vi "SSB.vi"() -> ()   [LabVIEW 2018]
uses:
  <vilib>/express/express analysis/Spectral/Block/exnSpectralBlock spectral measurements RMS poly.vi
  <vilib>/express/express analysis/Spectral/Block/exnSpectralBlock spectral measurements RMS DDT.vi
  <vilib>/express/express analysis/Spectral/XNode/ExpressSpectralMeasurementsBlockNode.xnode
panel:
  out "USB 2":dynamicdata(graph)
  out "Waveform Graph":dynamicdata(graph)
  out "LSB 2":dynamicdata(graph)
  out "USB":dynamicdata(graph)
  out "LSB":dynamicdata(graph)
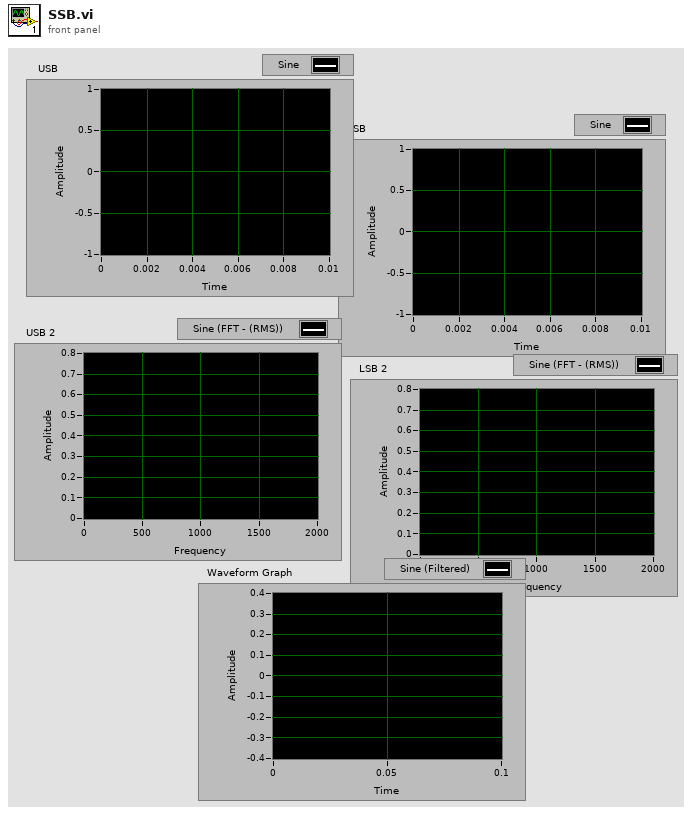
[diagram p1: front panel]
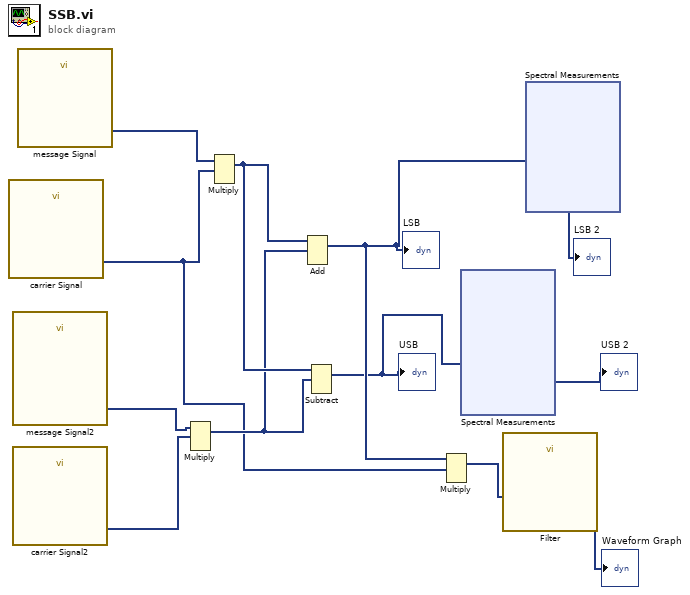
[diagram p0: block diagram]
diagram:
  n1 = call "carrier Signal"() -> ("Sine"=w7:dynamicdata)  [unwired: 14 in, 1 out]
  n2 = call "message Signal2"() -> ("Sine"=w11:dynamicdata)  [unwired: 14 in, 1 out]
  n3 = call "carrier Signal2"() -> ("Sine"=w10:dynamicdata)  [unwired: 14 in, 1 out]
  n4 = call "message Signal"() -> ("Sine"=w12:dynamicdata)  [unwired: 14 in, 1 out]
  n5 = Multiply(1:w10, 2:w11) -> (0:w8:dynamicdata)  [unwired: 1 in, 1 out]
  n6 = Multiply(1:w7, 2:w12) -> (0:w9:dynamicdata)  [unwired: 1 in, 1 out]
  n7 = Add(1:w8, 2:w9) -> (0:w5:dynamicdata)  [unwired: 1 in, 1 out]
  "LSB" <- w5
  n8 = Subtract(1:w8, 2:w9) -> (0:w2:dynamicdata)  [unwired: 1 in, 1 out]
  "USB" <- w2
  n9 = Multiply(1:w7, 2:w5) -> (0:w6:dynamicdata)  [unwired: 1 in, 1 out]
  n10 = xnode "Spectral Measurements"("Signals"=w2) -> ("FFT - (RMS)"=→"USB 2":dynamicdata)  [unwired: 1 in, 2 out]
  n11 = call "Filter"("Signal"=w6) -> ("Filtered Signal"=→"Waveform Graph":dynamicdata)  [unwired: 9 in, 1 out]
  n12 = xnode "Spectral Measurements"("Signals"=w5) -> ("FFT - (RMS)"=→"LSB 2":dynamicdata)  [unwired: 1 in, 2 out]
